vi "Delay.vi"(8 "Error In":errorcluster, 11 "Milliseconds To Wait":u32=100) -> (0 "Error Out":errorcluster)   [LabVIEW 2019, in "Utilities.lvlib"]
uses:
  Utilities.lvlib
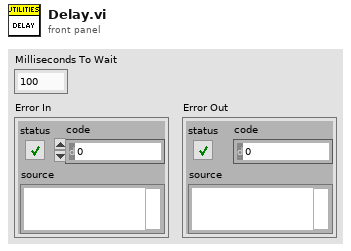
[diagram p1: front panel]
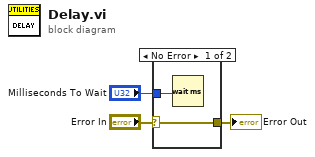
[diagram p0: block diagram]
diagram:
  n1 = case shown="No Error" "Error In" {
    selector: "Error In" -> [w5 w6]
    tunnel: [w5 w6] -> w2
    tunnel: "Milliseconds To Wait" -> [w4 _]
    frame No Error {
      n2 = Wait (ms)(milliseconds to wait=w4) -> ()  [unwired: 1 out]
    }
    frame Error {
    }
  }
  "Error Out" <- w2
